vi "simulator.vi"() -> ()   [LabVIEW 2013]
uses:
  control_type_defs.llb/rx_hw params.ctl
  control_type_defs.llb/rx_modulation params.ctl
  control_type_defs.llb/tx_hw params.ctl
  control_type_defs.llb/tx_modulation params.ctl
  control_type_defs.llb/tx_channel model params.ctl
  <vilib>/Analysis/baseanly.llb/Mean (DBL).vi
  <vilib>/measure/maspectr.llb/FFT Spectrum (Mag-Phase) for 1 Chan.vi
  <vilib>/Analysis/NI_AALBase.lvlib
  <vilib>/measure/NI_MAPro.lvlib
panel:
  in  "Matched Filtering parameters":T1={"modulation type"=enum."PSK", "pulse shaping filter"=enum."Raised Cosine", "filter parameter"=0.5, "filter length (symbols)"=8}
  out "error statistic":dbl format="%0.6f"
  out "estimated offset":i32
  out "average BER":dbl format="%0.6f"
  in  "Iterations":i32=1
  in  "packet length (bits)":i32=500
  in  "pulse shaping parameters":T1={"modulation type"=enum."PSK", "pulse shaping filter"=enum."Raised Cosine", "filter parameter"=0.5, "filter length (symbols)"=8}
  in  "control information for \npacket header/tail":T2={"Zero Pad Length"=8, "Training Sequence Type"="Barker Sequence-11"}
  in  "modulation type":string(combo)="QPSK"
  in  "Tab Control":T3(tab)
  out "Received Constellation":cluster{dbl[], dbl[]}(graph)
  out "Eye Diagram":cluster{"t0":dbl, "dt":dbl, "Y":dbl[]}[](graph)
  out "I Data":waveform(dbl)(graph)
  out "Q Data":waveform(dbl)(graph)
  out "Spectrum":cluster{"f0":dbl, "df":dbl, "magnitude":dbl[]}(graph)
  out "Spectrum 2":cluster{"f0":dbl, "df":dbl, "magnitude":dbl[]}(graph)
  out "Power Delay Profile":waveform(dbl)(graph)
  out "Measured channel impairements":T4
  in  "TX oversample factor":i32=4
  in  "TX sample rate":dbl(ring)=4000000.0 items=["100M"=100000000.0, "50M"=50000000.0, "33.3333M"=33333333.333333332, "25M"=25000000.0, "20M"=20000000.0, "16.6667M"=16666666.666666666, "14.2857M"=14285714.285714285, "12.5M"=12500000.0, "11.1111M"=11111111.111111112, "10M"=10000000.0, "9.09091M"=9090909.090909092, "8.33333M"=8333333.333333333, "7.69231M"=7692307.692307692, "7.14286M"=7142857.142857143, "6.66667M"=6666666.666666667, "6.25M"=6250000.0, "5.88235M"=5882352.94117647, "5.55556M"=5555555.555555556, "5.26316M"=5263157.894736842, "5M"=5000000.0, "4.7619M"=4761904.761904762, "4.54545M"=4545454.545454546, "4.34783M"=4347826.0869565215, "4.16667M"=4166666.6666666665, "4M"=4000000.0, "3.84615M"=3846153.846153846, "3.7037M"=3703703.703703704, "3.57143M"=3571428.5714285714, "3.44828M"=3448275.8620689656, "3.33333M"=3333333.3333333335, "3.22581M"=3225806.4516129033, "3.125M"=3125000.0, "3.0303M"=3030303.0303030303, "2.94118M"=2941176.470588235, "2.85714M"=2857142.8571428573, "2.77778M"=2777777.777777778, "2.7027M"=2702702.7027027025, "2.63158M"=2631578.947368421, "2.5641M"=2564102.564102564, "2.5M"=2500000.0, "2.43902M"=2439024.3902439023, "2.38095M"=2380952.380952381, "2.32558M"=2325581.395348837, "2.27273M"=2272727.272727273, "2.22222M"=2222222.222222222, "2.17391M"=2173913.0434782607, "2.12766M"=2127659.574468085, "2.08333M"=2083333.3333333333, "2.04082M"=2040816.3265306123, "2M"=2000000.0, "1.96078M"=1960784.3137254901, "1.92308M"=1923076.923076923, "1.88679M"=1886792.4528301887, "1.85185M"=1851851.851851852, "1.81818M"=1818181.8181818181, "1.78571M"=1785714.2857142857, "1.75439M"=1754385.9649122807, "1.72414M"=1724137.9310344828, "1.69492M"=1694915.2542372881, "1.66667M"=1666666.6666666667, "1.63934M"=1639344.262295082, "1.6129M"=1612903.2258064516, "1.5873M"=1587301.5873015872, "1.5625M"=1562500.0, "1.53846M"=1538461.5384615385, "1.51515M"=1515151.5151515151, "1.49254M"=1492537.3134328357, "1.47059M"=1470588.2352941176, "1.44928M"=1449275.3623188406, "1.42857M"=1428571.4285714286, "1.40845M"=1408450.704225352, "1.38889M"=1388888.888888889, "1.36986M"=1369863.01369863, "1.35135M"=1351351.3513513512, "1.33333M"=1333333.3333333333, "1.31579M"=1315789.4736842106, "1.2987M"=1298701.2987012987, "1.28205M"=1282051.282051282, "1.26582M"=1265822.7848101265, "1.25M"=1250000.0, "1.23457M"=1234567.9012345679, "1.21951M"=1219512.1951219512, "1.20482M"=1204819.2771084337, "1.19048M"=1190476.1904761905, "1.17647M"=1176470.5882352942, "1.16279M"=1162790.6976744186, "1.14943M"=1149425.287356322, "1.13636M"=1136363.6363636365, "1.1236M"=1123595.5056179776, "1.11111M"=1111111.111111111, "1.0989M"=1098901.0989010988, "1.08696M"=1086956.5217391304, "1.07527M"=1075268.817204301, "1.06383M"=1063829.7872340425, "1.05263M"=1052631.5789473683, "1.04167M"=1041666.6666666666, "1.03093M"=1030927.8350515463, "1.02041M"=1020408.1632653062, "1.0101M"=1010101.0101010101, "1M"=1000000.0, "990.099k"=990099.0099009901, "980.392k"=980392.1568627451, "970.874k"=970873.786407767, "961.538k"=961538.4615384615, "952.381k"=952380.9523809524, "943.396k"=943396.2264150943, "934.579k"=934579.4392523364, "925.926k"=925925.925925926, "917.431k"=917431.1926605505, "909.091k"=909090.9090909091, "900.901k"=900900.900900901, "892.857k"=892857.1428571428, "884.956k"=884955.7522123894, "877.193k"=877192.9824561403, "869.565k"=869565.2173913043, "862.069k"=862068.9655172414, "854.701k"=854700.8547008547, "847.458k"=847457.6271186441, "840.336k"=840336.1344537815, "833.333k"=833333.3333333334, "826.446k"=826446.2809917355, "819.672k"=819672.131147541, "813.008k"=813008.1300813009, "806.452k"=806451.6129032258, "800k"=800000.0, "793.651k"=793650.7936507936, "787.402k"=787401.5748031496, "781.25k"=781250.0, "769.231k"=769230.7692307692, "757.576k"=757575.7575757576, "746.269k"=746268.6567164179, "735.294k"=735294.1176470588, "724.638k"=724637.6811594203, "714.286k"=714285.7142857143, "704.225k"=704225.352112676, "694.444k"=694444.4444444445, "684.932k"=684931.506849315, "675.676k"=675675.6756756756, "666.667k"=666666.6666666666, "657.895k"=657894.7368421053, "649.351k"=649350.6493506493, "641.026k"=641025.641025641, "632.911k"=632911.3924050633, "625k"=625000.0, "617.284k"=617283.9506172839, "609.756k"=609756.0975609756, "602.41k"=602409.6385542168, "595.238k"=595238.0952380953, "588.235k"=588235.2941176471, "581.395k"=581395.3488372093, "574.713k"=574712.643678161, "568.182k"=568181.8181818182, "561.798k"=561797.7528089888, "555.556k"=555555.5555555555, "549.451k"=549450.5494505494, "543.478k"=543478.2608695652, "537.634k"=537634.4086021505, "531.915k"=531914.8936170213, "526.316k"=526315.7894736842, "520.833k"=520833.3333333333, "515.464k"=515463.91752577317, "510.204k"=510204.0816326531, "505.051k"=505050.50505050505, "500k"=500000.0, "495.05k"=495049.50495049503, "490.196k"=490196.07843137253, "485.437k"=485436.8932038835, "480.769k"=480769.23076923075, "476.19k"=476190.4761904762, "471.698k"=471698.11320754717, "467.29k"=467289.7196261682, "462.963k"=462962.962962963, "458.716k"=458715.59633027524, "454.545k"=454545.45454545453, "450.45k"=450450.4504504505, "446.429k"=446428.5714285714, "442.478k"=442477.8761061947, "438.596k"=438596.49122807017, "434.783k"=434782.60869565216, "431.034k"=431034.4827586207, "427.35k"=427350.4273504274, "423.729k"=423728.81355932204, "420.168k"=420168.06722689077, "416.667k"=416666.6666666667, "413.223k"=413223.14049586776, "409.836k"=409836.0655737705, "406.504k"=406504.0650406504, "403.226k"=403225.8064516129, "400k"=400000.0, "396.825k"=396825.3968253968, "393.701k"=393700.7874015748, "390.625k"=390625.0, "384.615k"=384615.3846153846, "378.788k"=378787.8787878788, "373.134k"=373134.32835820894, "367.647k"=367647.0588235294, "362.319k"=362318.84057971014, "357.143k"=357142.85714285716, "352.113k"=352112.676056338, "347.222k"=347222.22222222225, "342.466k"=342465.7534246575, "337.838k"=337837.8378378378, "333.333k"=333333.3333333333, "328.947k"=328947.36842105264, "324.675k"=324675.32467532466, "320.513k"=320512.8205128205, "316.456k"=316455.69620253163, "312.5k"=312500.0, "308.642k"=308641.97530864197, "304.878k"=304878.0487804878, "301.205k"=301204.8192771084, "297.619k"=297619.04761904763, "294.118k"=294117.64705882355, "290.698k"=290697.67441860464, "287.356k"=287356.3218390805, "284.091k"=284090.9090909091, "280.899k"=280898.8764044944, "277.778k"=277777.77777777775, "274.725k"=274725.2747252747, "271.739k"=271739.1304347826, "268.817k"=268817.20430107525, "265.957k"=265957.44680851063, "263.158k"=263157.8947368421, "260.417k"=260416.66666666666, "257.732k"=257731.95876288658, "255.102k"=255102.04081632654, "252.525k"=252525.25252525252, "250k"=250000.0, "247.525k"=247524.75247524751, "245.098k"=245098.03921568627, "242.718k"=242718.44660194175, "240.385k"=240384.61538461538, "238.095k"=238095.2380952381, "235.849k"=235849.05660377358, "233.645k"=233644.8598130841, "231.481k"=231481.4814814815, "229.358k"=229357.79816513762, "227.273k"=227272.72727272726, "225.225k"=225225.22522522524, "223.214k"=223214.2857142857, "221.239k"=221238.93805309734, "219.298k"=219298.24561403508, "217.391k"=217391.30434782608, "215.517k"=215517.24137931035, "213.675k"=213675.2136752137, "211.864k"=211864.40677966102, "210.084k"=210084.03361344538, "208.333k"=208333.33333333334, "206.612k"=206611.57024793388, "204.918k"=204918.03278688525, "203.252k"=203252.0325203252, "201.613k"=201612.90322580645, "200k"=200000.0, "198.413k"=198412.6984126984, "196.85k"=196850.3937007874, "195.312k"=195312.5]
  in  "RX Sample Rate":dbl(ring)=4000000.0 items=["100M"=100000000.0, "50M"=50000000.0, "33.3333M"=33333333.333333332, "25M"=25000000.0, "20M"=20000000.0, "16.6667M"=16666666.666666666, "14.2857M"=14285714.285714285, "12.5M"=12500000.0, "11.1111M"=11111111.111111112, "10M"=10000000.0, "9.09091M"=9090909.090909092, "8.33333M"=8333333.333333333, "7.69231M"=7692307.692307692, "7.14286M"=7142857.142857143, "6.66667M"=6666666.666666667, "6.25M"=6250000.0, "5.88235M"=5882352.94117647, "5.55556M"=5555555.555555556, "5.26316M"=5263157.894736842, "5M"=5000000.0, "4.7619M"=4761904.761904762, "4.54545M"=4545454.545454546, "4.34783M"=4347826.0869565215, "4.16667M"=4166666.6666666665, "4M"=4000000.0, "3.84615M"=3846153.846153846, "3.7037M"=3703703.703703704, "3.57143M"=3571428.5714285714, "3.44828M"=3448275.8620689656, "3.33333M"=3333333.3333333335, "3.22581M"=3225806.4516129033, "3.125M"=3125000.0, "3.0303M"=3030303.0303030303, "2.94118M"=2941176.470588235, "2.85714M"=2857142.8571428573, "2.77778M"=2777777.777777778, "2.7027M"=2702702.7027027025, "2.63158M"=2631578.947368421, "2.5641M"=2564102.564102564, "2.5M"=2500000.0, "2.43902M"=2439024.3902439023, "2.38095M"=2380952.380952381, "2.32558M"=2325581.395348837, "2.27273M"=2272727.272727273, "2.22222M"=2222222.222222222, "2.17391M"=2173913.0434782607, "2.12766M"=2127659.574468085, "2.08333M"=2083333.3333333333, "2.04082M"=2040816.3265306123, "2M"=2000000.0, "1.96078M"=1960784.3137254901, "1.92308M"=1923076.923076923, "1.88679M"=1886792.4528301887, "1.85185M"=1851851.851851852, "1.81818M"=1818181.8181818181, "1.78571M"=1785714.2857142857, "1.75439M"=1754385.9649122807, "1.72414M"=1724137.9310344828, "1.69492M"=1694915.2542372881, "1.66667M"=1666666.6666666667, "1.63934M"=1639344.262295082, "1.6129M"=1612903.2258064516, "1.5873M"=1587301.5873015872, "1.5625M"=1562500.0, "1.53846M"=1538461.5384615385, "1.51515M"=1515151.5151515151, "1.49254M"=1492537.3134328357, "1.47059M"=1470588.2352941176, "1.44928M"=1449275.3623188406, "1.42857M"=1428571.4285714286, "1.40845M"=1408450.704225352, "1.38889M"=1388888.888888889, "1.36986M"=1369863.01369863, "1.35135M"=1351351.3513513512, "1.33333M"=1333333.3333333333, "1.31579M"=1315789.4736842106, "1.2987M"=1298701.2987012987, "1.28205M"=1282051.282051282, "1.26582M"=1265822.7848101265, "1.25M"=1250000.0, "1.23457M"=1234567.9012345679, "1.21951M"=1219512.1951219512, "1.20482M"=1204819.2771084337, "1.19048M"=1190476.1904761905, "1.17647M"=1176470.5882352942, "1.16279M"=1162790.6976744186, "1.14943M"=1149425.287356322, "1.13636M"=1136363.6363636365, "1.1236M"=1123595.5056179776, "1.11111M"=1111111.111111111, "1.0989M"=1098901.0989010988, "1.08696M"=1086956.5217391304, "1.07527M"=1075268.817204301, "1.06383M"=1063829.7872340425, "1.05263M"=1052631.5789473683, "1.04167M"=1041666.6666666666, "1.03093M"=1030927.8350515463, "1.02041M"=1020408.1632653062, "1.0101M"=1010101.0101010101, "1M"=1000000.0, "990.099k"=990099.0099009901, "980.392k"=980392.1568627451, "970.874k"=970873.786407767, "961.538k"=961538.4615384615, "952.381k"=952380.9523809524, "943.396k"=943396.2264150943, "934.579k"=934579.4392523364, "925.926k"=925925.925925926, "917.431k"=917431.1926605505, "909.091k"=909090.9090909091, "900.901k"=900900.900900901, "892.857k"=892857.1428571428, "884.956k"=884955.7522123894, "877.193k"=877192.9824561403, "869.565k"=869565.2173913043, "862.069k"=862068.9655172414, "854.701k"=854700.8547008547, "847.458k"=847457.6271186441, "840.336k"=840336.1344537815, "833.333k"=833333.3333333334, "826.446k"=826446.2809917355, "819.672k"=819672.131147541, "813.008k"=813008.1300813009, "806.452k"=806451.6129032258, "800k"=800000.0, "793.651k"=793650.7936507936, "787.402k"=787401.5748031496, "781.25k"=781250.0, "769.231k"=769230.7692307692, "757.576k"=757575.7575757576, "746.269k"=746268.6567164179, "735.294k"=735294.1176470588, "724.638k"=724637.6811594203, "714.286k"=714285.7142857143, "704.225k"=704225.352112676, "694.444k"=694444.4444444445, "684.932k"=684931.506849315, "675.676k"=675675.6756756756, "666.667k"=666666.6666666666, "657.895k"=657894.7368421053, "649.351k"=649350.6493506493, "641.026k"=641025.641025641, "632.911k"=632911.3924050633, "625k"=625000.0, "617.284k"=617283.9506172839, "609.756k"=609756.0975609756, "602.41k"=602409.6385542168, "595.238k"=595238.0952380953, "588.235k"=588235.2941176471, "581.395k"=581395.3488372093, "574.713k"=574712.643678161, "568.182k"=568181.8181818182, "561.798k"=561797.7528089888, "555.556k"=555555.5555555555, "549.451k"=549450.5494505494, "543.478k"=543478.2608695652, "537.634k"=537634.4086021505, "531.915k"=531914.8936170213, "526.316k"=526315.7894736842, "520.833k"=520833.3333333333, "515.464k"=515463.91752577317, "510.204k"=510204.0816326531, "505.051k"=505050.50505050505, "500k"=500000.0, "495.05k"=495049.50495049503, "490.196k"=490196.07843137253, "485.437k"=485436.8932038835, "480.769k"=480769.23076923075, "476.19k"=476190.4761904762, "471.698k"=471698.11320754717, "467.29k"=467289.7196261682, "462.963k"=462962.962962963, "458.716k"=458715.59633027524, "454.545k"=454545.45454545453, "450.45k"=450450.4504504505, "446.429k"=446428.5714285714, "442.478k"=442477.8761061947, "438.596k"=438596.49122807017, "434.783k"=434782.60869565216, "431.034k"=431034.4827586207, "427.35k"=427350.4273504274, "423.729k"=423728.81355932204, "420.168k"=420168.06722689077, "416.667k"=416666.6666666667, "413.223k"=413223.14049586776, "409.836k"=409836.0655737705, "406.504k"=406504.0650406504, "403.226k"=403225.8064516129, "400k"=400000.0, "396.825k"=396825.3968253968, "393.701k"=393700.7874015748, "390.625k"=390625.0, "384.615k"=384615.3846153846, "378.788k"=378787.8787878788, "373.134k"=373134.32835820894, "367.647k"=367647.0588235294, "362.319k"=362318.84057971014, "357.143k"=357142.85714285716, "352.113k"=352112.676056338, "347.222k"=347222.22222222225, "342.466k"=342465.7534246575, "337.838k"=337837.8378378378, "333.333k"=333333.3333333333, "328.947k"=328947.36842105264, "324.675k"=324675.32467532466, "320.513k"=320512.8205128205, "316.456k"=316455.69620253163, "312.5k"=312500.0, "308.642k"=308641.97530864197, "304.878k"=304878.0487804878, "301.205k"=301204.8192771084, "297.619k"=297619.04761904763, "294.118k"=294117.64705882355, "290.698k"=290697.67441860464, "287.356k"=287356.3218390805, "284.091k"=284090.9090909091, "280.899k"=280898.8764044944, "277.778k"=277777.77777777775, "274.725k"=274725.2747252747, "271.739k"=271739.1304347826, "268.817k"=268817.20430107525, "265.957k"=265957.44680851063, "263.158k"=263157.8947368421, "260.417k"=260416.66666666666, "257.732k"=257731.95876288658, "255.102k"=255102.04081632654, "252.525k"=252525.25252525252, "250k"=250000.0, "247.525k"=247524.75247524751, "245.098k"=245098.03921568627, "242.718k"=242718.44660194175, "240.385k"=240384.61538461538, "238.095k"=238095.2380952381, "235.849k"=235849.05660377358, "233.645k"=233644.8598130841, "231.481k"=231481.4814814815, "229.358k"=229357.79816513762, "227.273k"=227272.72727272726, "225.225k"=225225.22522522524, "223.214k"=223214.2857142857, "221.239k"=221238.93805309734, "219.298k"=219298.24561403508, "217.391k"=217391.30434782608, "215.517k"=215517.24137931035, "213.675k"=213675.2136752137, "211.864k"=211864.40677966102, "210.084k"=210084.03361344538, "208.333k"=208333.33333333334, "206.612k"=206611.57024793388, "204.918k"=204918.03278688525, "203.252k"=203252.0325203252, "201.613k"=201612.90322580645, "200k"=200000.0, "198.413k"=198412.6984126984, "196.85k"=196850.3937007874, "195.312k"=195312.5]
  in  "RX oversample factor":i32=4
  in  "synchronization options":T5={"Symbol Timing Recovery Method"="Max Energy", "Synchronization Method"="Timing Estimation", "Correct Frequency Offset"=FALSE, "fixed offset"=0, "Frame Detection Method"="Sliding Correlator"}
  in  "channel estimation\nequalizer parameters":T6={"channel estimate length"=4, "equalizer length"=4, "equalizer delay"=-1, "Equalization Method"="Direct"}
  in  "TX channel model parameters":T7={"channel model"="AWGN", "noise power (dB)"=-inf, "channel response"=[], "frequency offset"=0.0, "delay (sec)"=0.0}
  out "error out":errorcluster
  in  "RX HW parameters":T8={"Device IP Address"="192.168.11.3", "Active Antenna"="RF1", "Carrier Frequency (Hz)"=2400000000.0, "Gain (dB)"=10.0, "Trigger Level"=0.01, "Bandwidth (Hz)"=40000000.0, "Reference Position (%)"=10.0, "Capture Time (s)"=0.0033, "Simulate"=FALSE} {"Capture Time (s)" format="%.2p"; "Bandwidth (Hz)" format="%.2p"; "Trigger Level" format="%#.3p"; "Gain (dB)" format="%.2f"; "Carrier Frequency (Hz)" format="%.2p"}
  in  "RX modulation parameters":T9={"modulation type"="QPSK", "pulse shaping parameters"={"modulation type"=enum."PSK", "pulse shaping filter"=enum."Root Raised Cos", "filter parameter"=0.5, "filter length (symbols)"=8}, "control information for packet header/tail"={"Training Sequence (derived)"=[0.7071067811865475+0.7071067811865475i, 0.7071067811865475+0.7071067811865475i, 0.7071067811865475+0.7071067811865475i, -0.7071067811865475-0.7071067811865475i, -0.7071067811865475-0.7071067811865475i, -0.7071067811865475-0.7071067811865475i, 0.7071067811865475+0.7071067811865475i, -0.7071067811865475-0.7071067811865475i, -0.7071067811865475-0.7071067811865475i, 0.7071067811865475+0.7071067811865475i, -0.7071067811865475-0.7071067811865475i, 0.7071067811865475+0.7071067811865475i, 0.7071067811865475+0.7071067811865475i, 0.7071067811865475+0.7071067811865475i, -0.7071067811865475-0.7071067811865475i, -0.7071067811865475-0.7071067811865475i, -0.7071067811865475-0.7071067811865475i, 0.7071067811865475+0.7071067811865475i, -0.7071067811865475-0.7071067811865475i, -0.7071067811865475-0.7071067811865475i, 0.7071067811865475+0.7071067811865475i, -0.7071067811865475-0.7071067811865475i, 0.7071067811865475+0.7071067811865475i, 0.7071067811865475+0.7071067811865475i, 0.7071067811865475+0.7071067811865475i, -0.7071067811865475-0.7071067811865475i, -0.7071067811865475-0.7071067811865475i, -0.7071067811865475-0.7071067811865475i, 0.7071067811865475+0.7071067811865475i, -0.7071067811865475-0.7071067811865475i, -0.7071067811865475-0.7071067811865475i, 0.7071067811865475+0.7071067811865475i, -0.7071067811865475-0.7071067811865475i, 0.7071067811865475+0.7071067811865475i, 0.7071067811865475+0.7071067811865475i, 0.7071067811865475+0.7071067811865475i, -0.7071067811865475-0.7071067811865475i, -0.7071067811865475-0.7071067811865475i, -0.7071067811865475-0.7071067811865475i, 0.7071067811865475+0.7071067811865475i, -0.7071067811865475-0.7071067811865475i, -0.7071067811865475-0.7071067811865475i, 0.7071067811865475+0.7071067811865475i, -0.7071067811865475-0.7071067811865475i], "Zero Pad Length"=8}, "RX oversample factor"=20, "channel estimation/equalizer\nparameters"={"channel estimate length"=1, "equalizer length"=1, "equalizer delay"=-1, "Equalization Method"="Direct"}, "synchronization options"={"Symbol Timing Recovery Method"="Max Energy", "Synchronization Method"="Timing Estimation", "Correct Frequency Offset"=FALSE, "fixed offset"=0, "Frame Detection Method"="Sliding Correlator"}, "number of data symbols (derived)"=100, "RX Sample Rate"=4000000.0} {"RX Sample Rate" items=["25M"=25000000.0, "20M"=20000000.0, "16.6667M"=16666666.666667, "14.2857M"=14285714.285714, "12.5M"=12500000.0, "11.1111M"=11111111.111111, "10M"=10000000.0, "9.09091M"=9090909.090909, "8.33333M"=8333333.333333, "7.69231M"=7692307.692308, "7.14286M"=7142857.142857, "6.66667M"=6666666.666667, "6.25M"=6250000.0, "5.88235M"=5882352.941176, "5.55556M"=5555555.555556, "5.26316M"=5263157.894737, "5M"=5000000.0, "4.7619M"=4761904.761905, "4.54545M"=4545454.545455, "4.34783M"=4347826.086957, "4.16667M"=4166666.666667, "4M"=4000000.0, "3.84615M"=3846153.846154, "3.7037M"=3703703.703704, "3.57143M"=3571428.571429, "3.44828M"=3448275.862069, "3.33333M"=3333333.333333, "3.22581M"=3225806.451613, "3.125M"=3125000.0, "3.0303M"=3030303.030303, "2.94118M"=2941176.470588, "2.85714M"=2857142.857143, "2.77778M"=2777777.777778, "2.7027M"=2702702.702703, "2.63158M"=2631578.947368, "2.5641M"=2564102.564103, "2.5M"=2500000.0, "2.43902M"=2439024.390244, "2.38095M"=2380952.380952, "2.32558M"=2325581.395349, "2.27273M"=2272727.272727, "2.22222M"=2222222.222222, "2.17391M"=2173913.043478, "2.12766M"=2127659.574468, "2.08333M"=2083333.333333, "2.04082M"=2040816.326531, "2M"=2000000.0, "1.96078M"=1960784.313725, "1.92308M"=1923076.923077, "1.88679M"=1886792.45283, "1.85185M"=1851851.851852, "1.81818M"=1818181.818182, "1.78571M"=1785714.285714, "1.75439M"=1754385.964912, "1.72414M"=1724137.931034, "1.69492M"=1694915.254237, "1.66667M"=1666666.666667, "1.63934M"=1639344.262295, "1.6129M"=1612903.225806, "1.5873M"=1587301.587302, "1.5625M"=1562500.0, "1.53846M"=1538461.538462, "1.51515M"=1515151.515152, "1.49254M"=1492537.313433, "1.47059M"=1470588.235294, "1.44928M"=1449275.362319, "1.42857M"=1428571.428571, "1.40845M"=1408450.704225, "1.38889M"=1388888.888889, "1.36986M"=1369863.013699, "1.35135M"=1351351.351351, "1.33333M"=1333333.333333, "1.31579M"=1315789.473684, "1.2987M"=1298701.298701, "1.28205M"=1282051.282051, "1.26582M"=1265822.78481, "1.25M"=1250000.0, "1.23457M"=1234567.901235, "1.21951M"=1219512.195122, "1.20482M"=1204819.277108, "1.19048M"=1190476.190476, "1.17647M"=1176470.588235, "1.16279M"=1162790.697674, "1.14943M"=1149425.287356, "1.13636M"=1136363.636364, "1.1236M"=1123595.505618, "1.11111M"=1111111.111111, "1.0989M"=1098901.098901, "1.08696M"=1086956.521739, "1.07527M"=1075268.817204, "1.06383M"=1063829.787234, "1.05263M"=1052631.578947, "1.04167M"=1041666.666667, "1.03093M"=1030927.835052, "1.02041M"=1020408.163265, "1.0101M"=1010101.010101, "1M"=1000000.0, "990.099k"=990099.009901, "980.392k"=980392.156863, "970.874k"=970873.786408, "961.538k"=961538.461538, "952.381k"=952380.952381, "943.396k"=943396.226415, "934.579k"=934579.439252, "925.926k"=925925.925926, "917.431k"=917431.192661, "909.091k"=909090.909091, "900.901k"=900900.900901, "892.857k"=892857.142857, "884.956k"=884955.752212, "877.193k"=877192.982456, "869.565k"=869565.217391, "862.069k"=862068.965517, "854.701k"=854700.854701, "847.458k"=847457.627119, "840.336k"=840336.134454, "833.333k"=833333.333333, "826.446k"=826446.280992, "819.672k"=819672.131148, "813.008k"=813008.130081, "806.452k"=806451.612903, "800k"=800000.0, "793.651k"=793650.793651, "787.402k"=787401.574803, "781.25k"=781250.0, "769.231k"=769230.769231, "757.576k"=757575.757576, "746.269k"=746268.656716, "735.294k"=735294.117647, "724.638k"=724637.681159, "714.286k"=714285.714286, "704.225k"=704225.352113, "694.444k"=694444.444444, "684.932k"=684931.506849, "675.676k"=675675.675676, "666.667k"=666666.666667, "657.895k"=657894.736842, "649.351k"=649350.649351, "641.026k"=641025.641026, "632.911k"=632911.392405, "625k"=625000.0, "617.284k"=617283.950617, "609.756k"=609756.097561, "602.41k"=602409.638554, "595.238k"=595238.095238, "588.235k"=588235.294118, "581.395k"=581395.348837, "574.713k"=574712.643678, "568.182k"=568181.818182, "561.798k"=561797.752809, "555.556k"=555555.555556, "549.451k"=549450.549451, "543.478k"=543478.26087, "537.634k"=537634.408602, "531.915k"=531914.893617, "526.316k"=526315.789474, "520.833k"=520833.333333, "515.464k"=515463.917526, "510.204k"=510204.081633, "505.051k"=505050.505051, "500k"=500000.0, "495.05k"=495049.50495, "490.196k"=490196.078431, "485.437k"=485436.893204, "480.769k"=480769.230769, "476.19k"=476190.47619, "471.698k"=471698.113208, "467.29k"=467289.719626, "462.963k"=462962.962963, "458.716k"=458715.59633, "454.545k"=454545.454545, "450.45k"=450450.45045, "446.429k"=446428.571429, "442.478k"=442477.876106, "438.596k"=438596.491228, "434.783k"=434782.608696, "431.034k"=431034.482759, "427.35k"=427350.42735, "423.729k"=423728.813559, "420.168k"=420168.067227, "416.667k"=416666.666667, "413.223k"=413223.140496, "409.836k"=409836.065574, "406.504k"=406504.065041, "403.226k"=403225.806452, "400k"=400000.0, "396.825k"=396825.396825, "393.701k"=393700.787402, "390.625k"=390625.0, "384.615k"=384615.384615, "378.788k"=378787.878788, "373.134k"=373134.328358, "367.647k"=367647.058824, "362.319k"=362318.84058, "357.143k"=357142.857143, "352.113k"=352112.676056, "347.222k"=347222.222222, "342.466k"=342465.753425, "337.838k"=337837.837838, "333.333k"=333333.333333, "328.947k"=328947.368421, "324.675k"=324675.324675, "320.513k"=320512.820513, "316.456k"=316455.696203, "312.5k"=312500.0, "308.642k"=308641.975309, "304.878k"=304878.04878, "301.205k"=301204.819277, "297.619k"=297619.047619, "294.118k"=294117.647059, "290.698k"=290697.674419, "287.356k"=287356.321839, "284.091k"=284090.909091, "280.899k"=280898.876404, "277.778k"=277777.777778, "274.725k"=274725.274725, "271.739k"=271739.130435, "268.817k"=268817.204301, "265.957k"=265957.446809, "263.158k"=263157.894737, "260.417k"=260416.666667, "257.732k"=257731.958763, "255.102k"=255102.040816, "252.525k"=252525.252525, "250k"=250000.0, "247.525k"=247524.752475, "245.098k"=245098.039216, "242.718k"=242718.446602, "240.385k"=240384.615385, "238.095k"=238095.238095, "235.849k"=235849.056604, "233.645k"=233644.859813, "231.481k"=231481.481481, "229.358k"=229357.798165, "227.273k"=227272.727273, "225.225k"=225225.225225, "223.214k"=223214.285714, "221.239k"=221238.938053, "219.298k"=219298.245614, "217.391k"=217391.304348, "215.517k"=215517.241379, "213.675k"=213675.213675, "211.864k"=211864.40678, "210.084k"=210084.033613, "208.333k"=208333.333333, "206.612k"=206611.570248, "204.918k"=204918.032787, "203.252k"=203252.03252, "201.613k"=201612.903226, "200k"=200000.0, "198.413k"=198412.698413, "196.85k"=196850.393701, "195.312k"=195312.5]; "control information for packet header/tail"."Training Sequence (derived)" format="%#_3p"}
  in  "TX HW parameters":T10={"Device IP Address"="192.168.11.3", "Active Antenna"="RF1", "Carrier Frequency (Hz)"=2400000000.0, "Gain (dB)"=10.0, "Generation Mode"=enum."single shot"} {"Gain (dB)" format="%.2f"; "Carrier Frequency (Hz)" format="%.2p"}
  in  "TX modulation parameters":T11={"modulation type"="QPSK", "pulse shaping parameters"={"modulation type"=enum."PSK", "pulse shaping filter"=enum."Root Raised Cos", "filter parameter"=0.5, "filter length (symbols)"=8}, "TX oversample factor"=20, "packet length (bits)"=500, "TX sample rate"=100.0, "control information for packet header/tail"={"Zero Pad Length"=8, "Training Sequence Type"="Barker Sequence-11"}} {"TX sample rate" items=["25M"=25000000.0, "20M"=20000000.0, "16.6667M"=16666666.666667, "14.2857M"=14285714.285714, "12.5M"=12500000.0, "11.1111M"=11111111.111111, "10M"=10000000.0, "9.09091M"=9090909.090909, "8.33333M"=8333333.333333, "7.69231M"=7692307.692308, "7.14286M"=7142857.142857, "6.66667M"=6666666.666667, "6.25M"=6250000.0, "5.88235M"=5882352.941176, "5.55556M"=5555555.555556, "5.26316M"=5263157.894737, "5M"=5000000.0, "4.7619M"=4761904.761905, "4.54545M"=4545454.545455, "4.34783M"=4347826.086957, "4.16667M"=4166666.666667, "4M"=4000000.0, "3.84615M"=3846153.846154, "3.7037M"=3703703.703704, "3.57143M"=3571428.571429, "3.44828M"=3448275.862069, "3.33333M"=3333333.333333, "3.22581M"=3225806.451613, "3.125M"=3125000.0, "3.0303M"=3030303.030303, "2.94118M"=2941176.470588, "2.85714M"=2857142.857143, "2.77778M"=2777777.777778, "2.7027M"=2702702.702703, "2.63158M"=2631578.947368, "2.5641M"=2564102.564103, "2.5M"=2500000.0, "2.43902M"=2439024.390244, "2.38095M"=2380952.380952, "2.32558M"=2325581.395349, "2.27273M"=2272727.272727, "2.22222M"=2222222.222222, "2.17391M"=2173913.043478, "2.12766M"=2127659.574468, "2.08333M"=2083333.333333, "2.04082M"=2040816.326531, "2M"=2000000.0, "1.96078M"=1960784.313725, "1.92308M"=1923076.923077, "1.88679M"=1886792.45283, "1.85185M"=1851851.851852, "1.81818M"=1818181.818182, "1.78571M"=1785714.285714, "1.75439M"=1754385.964912, "1.72414M"=1724137.931034, "1.69492M"=1694915.254237, "1.66667M"=1666666.666667, "1.63934M"=1639344.262295, "1.6129M"=1612903.225806, "1.5873M"=1587301.587302, "1.5625M"=1562500.0, "1.53846M"=1538461.538462, "1.51515M"=1515151.515152, "1.49254M"=1492537.313433, "1.47059M"=1470588.235294, "1.44928M"=1449275.362319, "1.42857M"=1428571.428571, "1.40845M"=1408450.704225, "1.38889M"=1388888.888889, "1.36986M"=1369863.013699, "1.35135M"=1351351.351351, "1.33333M"=1333333.333333, "1.31579M"=1315789.473684, "1.2987M"=1298701.298701, "1.28205M"=1282051.282051, "1.26582M"=1265822.78481, "1.25M"=1250000.0, "1.23457M"=1234567.901235, "1.21951M"=1219512.195122, "1.20482M"=1204819.277108, "1.19048M"=1190476.190476, "1.17647M"=1176470.588235, "1.16279M"=1162790.697674, "1.14943M"=1149425.287356, "1.13636M"=1136363.636364, "1.1236M"=1123595.505618, "1.11111M"=1111111.111111, "1.0989M"=1098901.098901, "1.08696M"=1086956.521739, "1.07527M"=1075268.817204, "1.06383M"=1063829.787234, "1.05263M"=1052631.578947, "1.04167M"=1041666.666667, "1.03093M"=1030927.835052, "1.02041M"=1020408.163265, "1.0101M"=1010101.010101, "1M"=1000000.0, "990.099k"=990099.009901, "980.392k"=980392.156863, "970.874k"=970873.786408, "961.538k"=961538.461538, "952.381k"=952380.952381, "943.396k"=943396.226415, "934.579k"=934579.439252, "925.926k"=925925.925926, "917.431k"=917431.192661, "909.091k"=909090.909091, "900.901k"=900900.900901, "892.857k"=892857.142857, "884.956k"=884955.752212, "877.193k"=877192.982456, "869.565k"=869565.217391, "862.069k"=862068.965517, "854.701k"=854700.854701, "847.458k"=847457.627119, "840.336k"=840336.134454, "833.333k"=833333.333333, "826.446k"=826446.280992, "819.672k"=819672.131148, "813.008k"=813008.130081, "806.452k"=806451.612903, "800k"=800000.0, "793.651k"=793650.793651, "787.402k"=787401.574803, "781.25k"=781250.0, "769.231k"=769230.769231, "757.576k"=757575.757576, "746.269k"=746268.656716, "735.294k"=735294.117647, "724.638k"=724637.681159, "714.286k"=714285.714286, "704.225k"=704225.352113, "694.444k"=694444.444444, "684.932k"=684931.506849, "675.676k"=675675.675676, "666.667k"=666666.666667, "657.895k"=657894.736842, "649.351k"=649350.649351, "641.026k"=641025.641026, "632.911k"=632911.392405, "625k"=625000.0, "617.284k"=617283.950617, "609.756k"=609756.097561, "602.41k"=602409.638554, "595.238k"=595238.095238, "588.235k"=588235.294118, "581.395k"=581395.348837, "574.713k"=574712.643678, "568.182k"=568181.818182, "561.798k"=561797.752809, "555.556k"=555555.555556, "549.451k"=549450.549451, "543.478k"=543478.26087, "537.634k"=537634.408602, "531.915k"=531914.893617, "526.316k"=526315.789474, "520.833k"=520833.333333, "515.464k"=515463.917526, "510.204k"=510204.081633, "505.051k"=505050.505051, "500k"=500000.0, "495.05k"=495049.50495, "490.196k"=490196.078431, "485.437k"=485436.893204, "480.769k"=480769.230769, "476.19k"=476190.47619, "471.698k"=471698.113208, "467.29k"=467289.719626, "462.963k"=462962.962963, "458.716k"=458715.59633, "454.545k"=454545.454545, "450.45k"=450450.45045, "446.429k"=446428.571429, "442.478k"=442477.876106, "438.596k"=438596.491228, "434.783k"=434782.608696, "431.034k"=431034.482759, "427.35k"=427350.42735, "423.729k"=423728.813559, "420.168k"=420168.067227, "416.667k"=416666.666667, "413.223k"=413223.140496, "409.836k"=409836.065574, "406.504k"=406504.065041, "403.226k"=403225.806452, "400k"=400000.0, "396.825k"=396825.396825, "393.701k"=393700.787402, "390.625k"=390625.0, "384.615k"=384615.384615, "378.788k"=378787.878788, "373.134k"=373134.328358, "367.647k"=367647.058824, "362.319k"=362318.84058, "357.143k"=357142.857143, "352.113k"=352112.676056, "347.222k"=347222.222222, "342.466k"=342465.753425, "337.838k"=337837.837838, "333.333k"=333333.333333, "328.947k"=328947.368421, "324.675k"=324675.324675, "320.513k"=320512.820513, "316.456k"=316455.696203, "312.5k"=312500.0, "308.642k"=308641.975309, "304.878k"=304878.04878, "301.205k"=301204.819277, "297.619k"=297619.047619, "294.118k"=294117.647059, "290.698k"=290697.674419, "287.356k"=287356.321839, "284.091k"=284090.909091, "280.899k"=280898.876404, "277.778k"=277777.777778, "274.725k"=274725.274725, "271.739k"=271739.130435, "268.817k"=268817.204301, "265.957k"=265957.446809, "263.158k"=263157.894737, "260.417k"=260416.666667, "257.732k"=257731.958763, "255.102k"=255102.040816, "252.525k"=252525.252525, "250k"=250000.0, "247.525k"=247524.752475, "245.098k"=245098.039216, "242.718k"=242718.446602, "240.385k"=240384.615385, "238.095k"=238095.238095, "235.849k"=235849.056604, "233.645k"=233644.859813, "231.481k"=231481.481481, "229.358k"=229357.798165, "227.273k"=227272.727273, "225.225k"=225225.225225, "223.214k"=223214.285714, "221.239k"=221238.938053, "219.298k"=219298.245614, "217.391k"=217391.304348, "215.517k"=215517.241379, "213.675k"=213675.213675, "211.864k"=211864.40678, "210.084k"=210084.033613, "208.333k"=208333.333333, "206.612k"=206611.570248, "204.918k"=204918.032787, "203.252k"=203252.03252, "201.613k"=201612.903226, "200k"=200000.0, "198.413k"=198412.698413, "196.85k"=196850.393701, "195.312k"=195312.5]}
  # "RECEIVER"
  # "TRANSMITTER"
  # "SHARED"
  # "( set delay to -1 for equalizer\n  to choose optimal delay )"
  # "( set delay to -1 for equalizer\n  to choose optimal delay )"
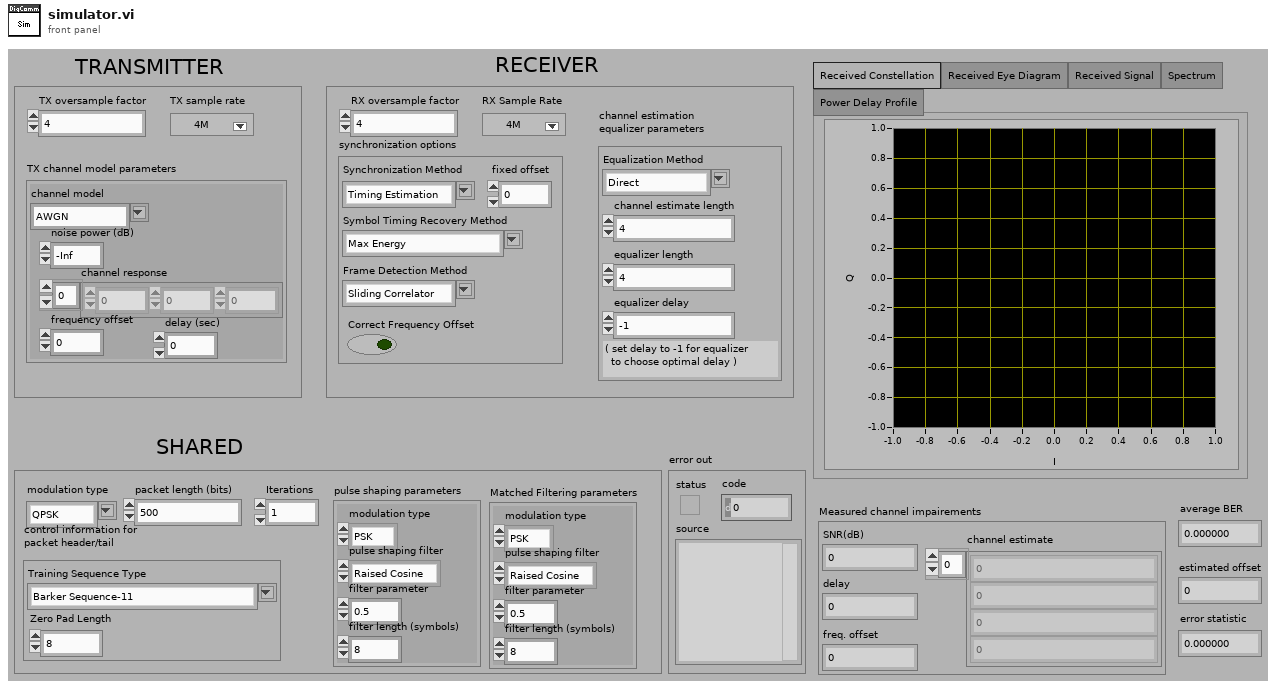
[diagram p1: front panel]
types:
  T1 = cluster{"modulation type":enum16{"FSK", "PSK", "QAM", "MSK", "PAM", "ASK"}, "pulse shaping filter":enum16{"none", "Raised Cosine", "Root Raised Cos", "Gaussian"}, "filter parameter":dbl, "filter length (symbols)":i32}
  T2 = cluster{"Zero Pad Length":i32, "Training Sequence Type":string}
  T3 = enum32{"Received Constellation", "Received Eye Diagram", "Received Signal", "Spectrum", "Power Delay Profile"}
  T4 = cluster{"SNR(dB)":dbl, "channel estimate":cdb[], "freq. offset":dbl, "delay":dbl}
  T5 = cluster{"Symbol Timing Recovery Method":string, "Synchronization Method":string, "Correct Frequency Offset":bool, "fixed offset":i32, "Frame Detection Method":string}
  T6 = cluster{"channel estimate length":i32, "equalizer length":i32, "equalizer delay":i32, "Equalization Method":string}
  T7 = typedef "tx_channel model params.ctl" = cluster{"channel model":string, "noise power (dB)":dbl, "channel response":cdb[], "frequency offset":dbl, "delay (sec)":dbl}
  T8 = typedef "rx_hw params.ctl" = cluster{"Device IP Address":refnum<k15>, "Active Antenna":string, "Carrier Frequency (Hz)":dbl, "Gain (dB)":dbl, "Trigger Level":dbl, "Bandwidth (Hz)":dbl, "Reference Position (%)":dbl, "Capture Time (s)":dbl, "Simulate":bool}
  T9 = typedef "rx_modulation params.ctl" = cluster{"modulation type":string, "pulse shaping parameters":cluster{"modulation type":enum16{"FSK", "PSK", "QAM", "MSK", "PAM", "ASK"}, "pulse shaping filter":enum16{"none", "Raised Cosine", "Root Raised Cos", "Gaussian"}, "filter parameter":dbl, "filter length (symbols)":i32}, "control information for packet header/tail":cluster{"Training Sequence (derived)":cdb[], "Zero Pad Length":i32}, "RX oversample factor":i32, "channel estimation/equalizer\nparameters":cluster{"channel estimate length":i32, "equalizer length":i32, "equalizer delay":i32, "Equalization Method":string}, "synchronization options":cluster{"Symbol Timing Recovery Method":string, "Synchronization Method":string, "Correct Frequency Offset":bool, "fixed offset":i32, "Frame Detection Method":string}, "number of data symbols (derived)":i32, "RX Sample Rate":dbl}
  T10 = typedef "tx_hw params.ctl" = cluster{"Device IP Address":refnum<k15>, "Active Antenna":string, "Carrier Frequency (Hz)":dbl, "Gain (dB)":dbl, "Generation Mode":enum16{"single shot", "simulate", "continuous"}}
  T11 = typedef "tx_modulation params.ctl" = cluster{"modulation type":string, "pulse shaping parameters":cluster{"modulation type":enum16{"FSK", "PSK", "QAM", "MSK", "PAM", "ASK"}, "pulse shaping filter":enum16{"none", "Raised Cosine", "Root Raised Cos", "Gaussian"}, "filter parameter":dbl, "filter length (symbols)":i32}, "TX oversample factor":i32, "packet length (bits)":i32, "TX sample rate":dbl, "control information for packet header/tail":cluster{"Zero Pad Length":i32, "Training Sequence Type":string}}
  T12 = cluster{"Training Sequence (derived)":cdb[], "Zero Pad Length":i32}
  T13 = cluster{"dB On (F)":bool, "unwrap phase (F)":bool, "convert to degree (F)":bool}
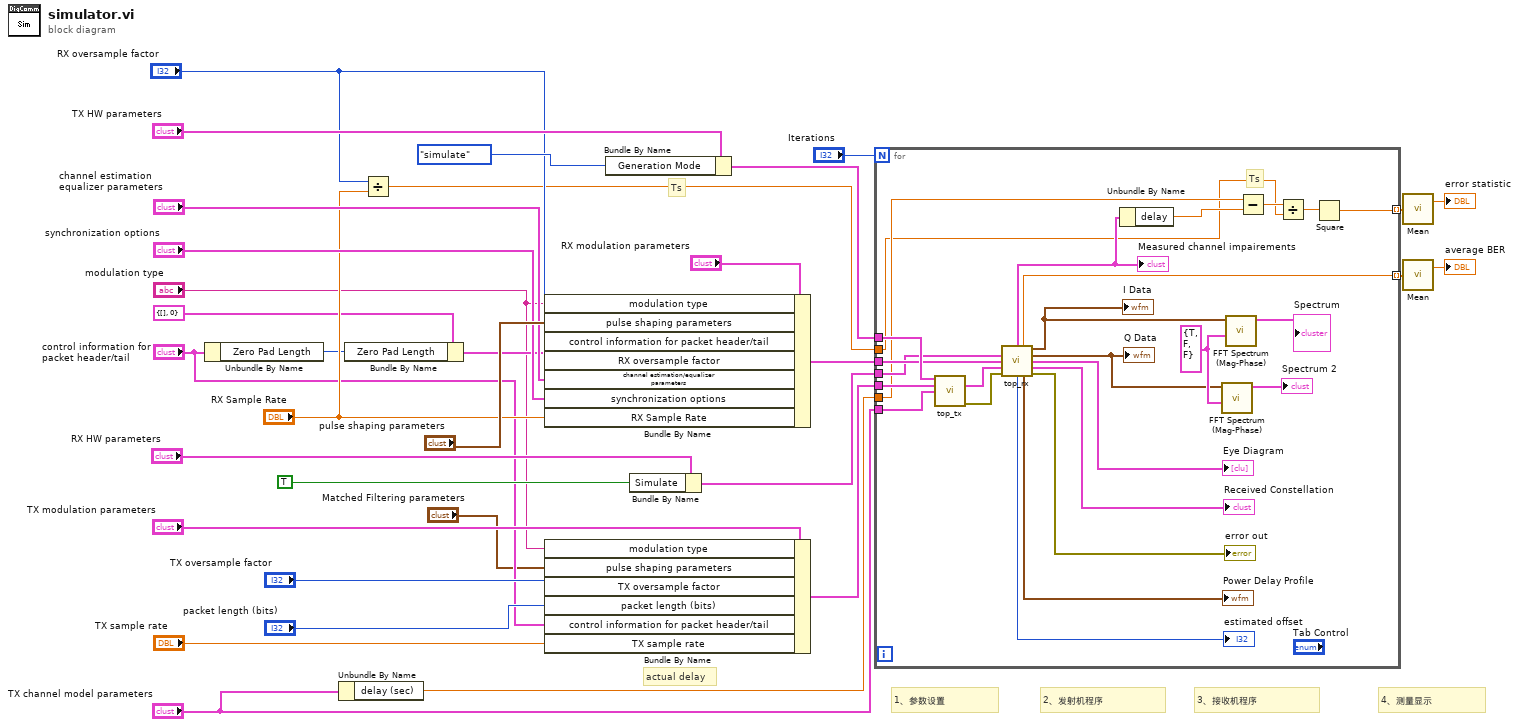
[diagram p0: block diagram]
diagram:
  # "4、测量显示"
  # "3、接收机程序"
  # "2、发射机程序"
  # "1、参数设置"
  # "actual delay"
  # "Ts"
  n1 = Unbundle By Name("control information for \npacket header/tail") -> ("Zero Pad Length"=w4:i32)
  n2 = Unbundle By Name("TX channel model parameters") -> ("delay (sec)"=w10:dbl)
  n3 = Bundle By Name(cluster=T12 {"Training Sequence (derived)"=[], "Zero Pad Length"=0} ("control information\nfor packet header/tail"), "Zero Pad Length"=w4) -> (w3:T12)
  n4 = Divide(x="RX oversample factor", y="RX Sample Rate") -> (x/y=w9:dbl)
  n5 = Bundle By Name(cluster="RX modulation parameters", "modulation type"="modulation type", "pulse shaping parameters"="pulse shaping parameters", "control information for packet header/tail"=w3, "RX oversample factor"="RX oversample factor", "channel estimation/equalizer\nparameters"="channel estimation\nequalizer parameters", "synchronization options"="synchronization options", "RX Sample Rate"="RX Sample Rate") -> (w19:T9)
  n6 = Bundle By Name(cluster="TX modulation parameters", "modulation type"="modulation type", "pulse shaping parameters"="Matched Filtering parameters", "TX oversample factor"="TX oversample factor", "packet length (bits)"="packet length (bits)", "control information for packet header/tail"="control information for \npacket header/tail", "TX sample rate"="TX sample rate") -> (w25:T11)
  n7 = Bundle By Name(cluster="TX HW parameters", "Generation Mode"=enum16{"single shot", "simulate", "continuous"}."simulate") -> (w30:T10)
  n8 = Bundle By Name(cluster="RX HW parameters", "Simulate"=TRUE) -> (w18:T8)
  n9 = for {
    N: "Iterations" -> [_]
    tunnel: "TX channel model parameters" -> [w57]
    tunnel: w30 -> [w56]
    tunnel: w25 -> [w55]
    tunnel: w19 -> [w54]
    tunnel: w18 -> [w53]
    tunnel: [w49] -> w16 mode=indexing
    tunnel: w10 -> [w42]
    tunnel: w9 -> [w40]
    tunnel: [w38] -> w8 mode=indexing
    w35 = T13 {"dB On (F)"=TRUE, "unwrap phase (F)"=FALSE, "convert to degree (F)"=FALSE} ("view")
    # "Ts"
    n10 = call "top_tx.vi"("HW parameters"=w56, "modulation parameters"=w55, "channel model parameters"=w57) -> ("output IQ waveform"=w47:cluster{"t0":dbl, "dt":dbl, "Y":cdb[]}, "error out"=w48:errorcluster)  [unwired: 8 in, 3 out]
    n11 = call "top_rx.vi"("HW parameters"=w53, "modulation parameters"=w54, "Received IQ\nwaveform"=w47, "error in"=w48) -> ("Measured channel impairements"=w44:T4, "average \nbit-error rate"=w49:dbl, "I Data"=w34:waveform(dbl), "Q Data"=w33:waveform(dbl), "Eye Diagram"=→"Eye Diagram":cluster{"t0":dbl, "dt":dbl, "Y":dbl[]}[], "Received\n Constellation"=→"Received Constellation":cluster{dbl[], dbl[]}, "offset"=→"estimated offset":i32, "Power Delay Profile"=→"Power Delay Profile":waveform(dbl), "error out"=→"error out":errorcluster)  [unwired: 3 in]
    "Measured channel impairements" <- w44
    "I Data" <- w34
    "Q Data" <- w33
    n12 = Unbundle By Name(w44) -> ("delay"=w41:dbl)
    n13 = call-poly <vilib>:"FFT Spectrum (Mag-Phase).vi"("view"=w35, "time signal"=w33) -> ("magnitude"=→"Spectrum 2":cluster{"f0":dbl, "df":dbl, "magnitude":dbl[]})  [unwired: 5 in, 4 out]
    n14 = call-poly <vilib>:"FFT Spectrum (Mag-Phase).vi"("view"=w35, "time signal"=w34) -> ("magnitude"=→"Spectrum":cluster{"f0":dbl, "df":dbl, "magnitude":dbl[]})  [unwired: 5 in, 4 out]
    n15 = Subtract(x=w42, y=w41) -> (x-y=w43:dbl)
    n16 = Divide(x=w43, y=w40) -> (x/y=w39:dbl)
    n17 = Square(x=w39) -> (x^2=w38:dbl)
  }
  n18 = call-poly <vilib>:"Mean.vi"("X"=w8) -> ("mean"=→"error statistic":dbl)  [unwired: 1 out]
  n19 = call-poly <vilib>:"Mean.vi"("X"=w16) -> ("mean"=→"average BER":dbl)  [unwired: 1 out]
